vi "Convert Sensor Values.vi"(11 "ECE Units":dbl[](array[numeric])) -> (3 "CBME Units":dbl[](array[numeric]))   [LabVIEW 2017]
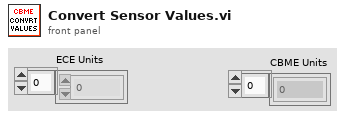
[diagram p1: front panel]
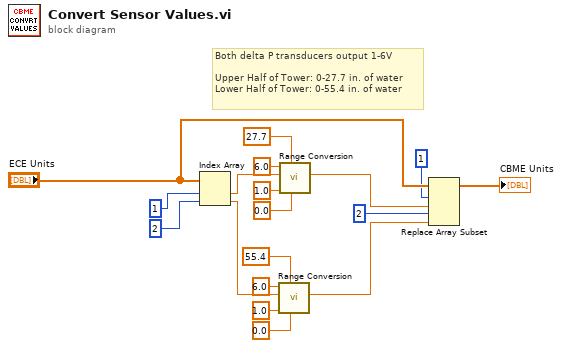
[diagram p0: block diagram]
diagram:
  # "Both delta P transducers output 1-6V\n\nUpper Half of Tower: 0-27.7 in. of water\nLower Half of Tower: 0-55.4 in. of water"
  n1 = Index Array(array="ECE Units", index #1=1 ("index"), index #2=2 ("index")) -> (element #1=w12:dbl, element #2=w6:dbl)
  n2 = call "Range Conversion.vi"("New Min"=0.0, "New Max"=55.4, "Current Min"=1.0, "Input Value"=w6, "Current Max"=6.0) -> ("Scaled Output"=w1:dbl)  [unwired: 6 in]
  n3 = call "Range Conversion.vi"("New Min"=0.0, "New Max"=27.7, "Current Min"=1.0, "Input Value"=w12, "Current Max"=6.0) -> ("Scaled Output"=w7:dbl)  [unwired: 6 in]
  n4 = Replace Array Subset(array="ECE Units", new element #1=w7, index #1=1 ("index"), new element #2=w1, index #2=2 ("index")) -> (→"CBME Units":dbl[])
